vi "setpoint and rotate.vi"(0 "axis 1: sp position °":dbl, 1 "m/c temp setpoint":dbl, 5 "move axis 1":bool, 7 "axis 2: sp position °":dbl, 9 "move axis 2":bool, 11 "error in":errorcluster) -> (4 "Status OUT":T1, 15 "error out":errorcluster)   [LabVIEW 2019]
uses:
  <vilib>/Analysis/NI_AALBase.lvlib
panel:
  out "iterations":i32
  out "standard deviation":dbl format="%0.2f"
  out "mean temperature":dbl format="%0.2f"
  out "m/c temp":dbl
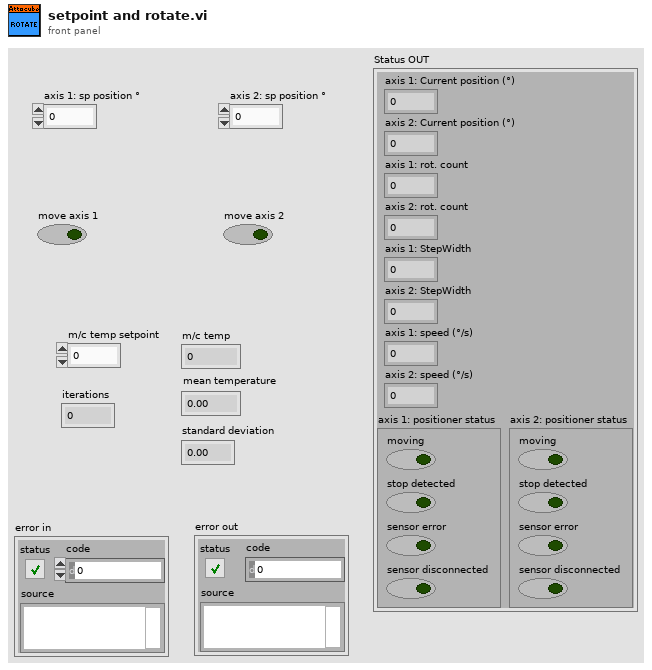
[diagram p1: front panel]
types:
  T1 = cluster{"axis 1: Current position (°)":dbl, "axis 2: Current position (°)":dbl, "axis 1: rot. count":dbl, "axis 2: rot. count":dbl, "axis 1: StepWidth":dbl, "axis 2: StepWidth":dbl, "axis 1: speed (°/s)":dbl, "axis 2: speed (°/s)":dbl, "axis 1: positioner status":cluster{"moving":bool, "stop detected":bool, "sensor error":bool, "sensor disconnected":bool}, "axis 2: positioner status":cluster{"moving":bool, "stop detected":bool, "sensor error":bool, "sensor disconnected":bool}}
  T2 = cluster{"axis 1: Absolute":bool, "axis 2: Absolute":bool, "axis 1: Stop moving":bool, "axis 2: Stop moving":bool, "axis 1: Output":bool, "axis 2: Output":bool, "set static amplitude\nwhen moving":bool}
  T3 = cluster{"axis 1: Amplitude [V]":dbl, "axis 2: Amplitude [V]":dbl, "axis 1: DCLevel [V]":dbl, "axis 2: DCLevel [V]":dbl, "axis 1: Frequency [Hz]":dbl, "axis 2: Frequency [Hz]":dbl, "axis 1: sp position °":dbl, "axis 2: sp position °":dbl, "axis 1: sp rot count":dbl, "axis 2: sp rot count":dbl}
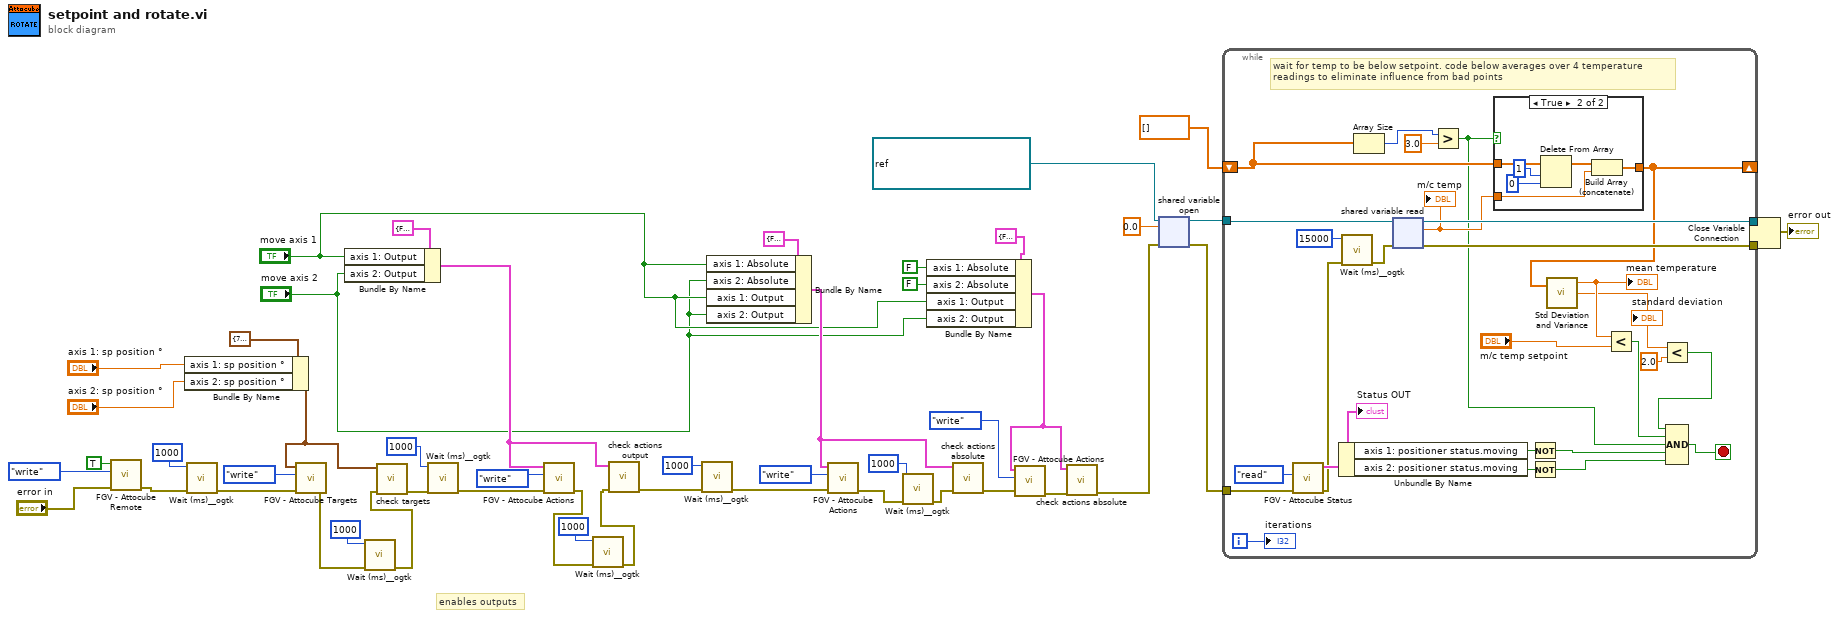
[diagram p0: block diagram]
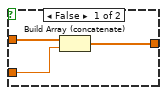
[diagram p2: hidden frame]
diagram:
  # "enables outputs"
  n1 = call "FGV - Attocube Remote.vi"("error in"="error in", "Function"=enum16{"write", "read"}."write", "Attocube Remote"=TRUE) -> ("error out"=w28:errorcluster)  [unwired: 3 in, 1 out]
  n2 = Bundle By Name(cluster=T3 {"axis 1: Amplitude [V]"=70.0, "axis 2: Amplitude [V]"=65.0, "axis 1: DCLevel [V]"=0.0, "axis 2: DCLevel [V]"=0.0, "axis 1: Frequency [Hz]"=3500.0, "axis 2: Frequency [Hz]"=3500.0, "axis 1: sp position °"=230.0, "axis 2: sp position °"=255.0, "axis 1: sp rot count"=0.0, "axis 2: sp rot count"=0.0} ("Targets In"), "axis 1: sp position °"="axis 1: sp position °", "axis 2: sp position °"="axis 2: sp position °") -> (w21:T3)
  n3 = call <userlib>:"Wait (ms)__ogtk.vi"("error in (no error)"=w28, "milliseconds to wait"=u32 1000) -> ("error out"=w27:errorcluster)  [unwired: 8 in, 1 out]
  n4 = call "FGV - Attocube Targets.vi"("error in"=w27, "Function"=enum16{"write", "read"}."write", "Targets In"=w21) -> ("error out"=w19:errorcluster)  [unwired: 3 in, 1 out]
  n5 = Bundle By Name(cluster=T2 {"axis 1: Absolute"=FALSE, "axis 2: Absolute"=FALSE, "axis 1: Stop moving"=FALSE, "axis 2: Stop moving"=FALSE, "axis 1: Output"=FALSE, "axis 2: Output"=FALSE, "set static amplitude\nwhen moving"=FALSE} ("Actions IN"), "axis 1: Output"="move axis 1", "axis 2: Output"="move axis 2") -> (w24:T2)
  n6 = call <userlib>:"Wait (ms)__ogtk.vi"("error in (no error)"=w19, "milliseconds to wait"=u32 1000) -> ("error out"=w18:errorcluster)  [unwired: 8 in, 1 out]
  n7 = call "check targets.vi"("error in"=w18, "Targets In"=w21) -> ("error in 2"=w25:errorcluster)  [unwired: 9 in]
  n8 = call <userlib>:"Wait (ms)__ogtk.vi"("error in (no error)"=w25, "milliseconds to wait"=u32 1000) -> ("error out"=w30:errorcluster)  [unwired: 8 in, 1 out]
  n9 = call "FGV - Attocube Actions.vi"("error in"=w30, "Function"=enum16{"write", "read"}."write", "Actions IN"=w24) -> ("error out"=w16:errorcluster)  [unwired: 3 in, 1 out]
  n10 = call <userlib>:"Wait (ms)__ogtk.vi"("error in (no error)"=w16, "milliseconds to wait"=u32 1000) -> ("error out"=w15:errorcluster)  [unwired: 8 in, 1 out]
  n11 = call "check actions output.vi"("error in"=w15, "Actions IN"=w24) -> ("error in 2"=w23:errorcluster)  [unwired: 9 in]
  n12 = call <userlib>:"Wait (ms)__ogtk.vi"("error in (no error)"=w23, "milliseconds to wait"=u32 1000) -> ("error out"=w32:errorcluster)  [unwired: 8 in, 1 out]
  n13 = Bundle By Name(cluster=T2 {"axis 1: Absolute"=FALSE, "axis 2: Absolute"=FALSE, "axis 1: Stop moving"=FALSE, "axis 2: Stop moving"=FALSE, "axis 1: Output"=FALSE, "axis 2: Output"=FALSE, "set static amplitude\nwhen moving"=FALSE} ("Actions IN"), "axis 1: Absolute"="move axis 1", "axis 2: Absolute"="move axis 2", "axis 1: Output"="move axis 1", "axis 2: Output"="move axis 2") -> (w22:T2)
  n14 = call "FGV - Attocube Actions.vi"("error in"=w32, "Function"=enum16{"write", "read"}."write", "Actions IN"=w22) -> ("error out"=w12:errorcluster)  [unwired: 3 in, 1 out]
  n15 = call <userlib>:"Wait (ms)__ogtk.vi"("error in (no error)"=w12, "milliseconds to wait"=u32 1000) -> ("error out"=w14:errorcluster)  [unwired: 8 in, 1 out]
  n16 = Bundle By Name(cluster=T2 {"axis 1: Absolute"=FALSE, "axis 2: Absolute"=FALSE, "axis 1: Stop moving"=FALSE, "axis 2: Stop moving"=FALSE, "axis 1: Output"=FALSE, "axis 2: Output"=FALSE, "set static amplitude\nwhen moving"=FALSE} ("Actions IN"), "axis 1: Absolute"=FALSE, "axis 2: Absolute"=FALSE, "axis 1: Output"="move axis 1", "axis 2: Output"="move axis 2") -> (w2:T2)
  n17 = call "check actions absolute.vi"("error in"=w14, "Actions IN"=w22) -> ("error in 2"=w11:errorcluster)  [unwired: 9 in]
  n18 = call "FGV - Attocube Actions.vi"("error in"=w11, "Function"=enum16{"write", "read"}."write", "Actions IN"=w2) -> ("error out"=w8:errorcluster)  [unwired: 3 in, 1 out]
  n19 = call "check actions absolute.vi"("error in"=w8, "Actions IN"=w2) -> ("error in 2"=w3:errorcluster)  [unwired: 9 in]
  n20 = shared-variable-open(refnum<k21> "ni.var.psp://housesoftheholy/MNK_18T/MNK_TC_T3" ("shared variable refnum in"), w3, 0.0) -> (w36:refnum<k21>, w37:errorcluster)  [unwired: 1 in]
  n21 = while {
    tunnel: w37 -> [w75]
    tunnel: w36 -> [w72]
    tunnel: [w71] -> w35
    tunnel: [w70] -> w34
    shift-right: [w61] -> _
    shift-left: dbl[] [] -> [w66]
    i -> [w51]
    stop <- w56 stop-if-true
    # "wait for temp to be below setpoint. code below averages over 4 temperature\nreadings to eliminate influence from bad points"
    n22 = call "FGV - Attocube Status.vi"("error in"=w75, "Function"=enum16{"write", "read"}."read") -> ("error out"=w67:errorcluster, "Status OUT"=w77:T1)  [unwired: 4 in]
    "Status OUT" <- w77
    n23 = Unbundle By Name(w77) -> ("axis 1: positioner status.moving"=w74:bool, "axis 2: positioner status.moving"=w73:bool)
    n24 = call <userlib>:"Wait (ms)__ogtk.vi"("error in (no error)"=w67, "milliseconds to wait"=u32 15000) -> ("error out"=w63:errorcluster)  [unwired: 8 in, 1 out]
    n25 = Array Size(array=w66) -> (size(s)=w64:i32)
    n26 = shared-variable-read(w72, w63) -> (w71:refnum<k21>, w70:errorcluster, w62:dbl)  [unwired: 1 out]
    "m/c temp" <- w62
    n27 = Greater?(x=w64, y=3.0) -> (0:w55:bool)
    n28 = case shown="True" w55 {
      tunnel: w66 -> [w80 w86]
      tunnel: [w79 w81] -> w61
      tunnel: w62 -> [w78 w82]
      frame False {
        n29 = Build Array (concatenate)(w80, w78) -> (w79:dbl[])
      }
      frame True {
        n30 = Delete From Array(array=w86, length=1, index=0) -> (array with subset deleted=w83:dbl[])  [unwired: 1 out]
        n31 = Build Array (concatenate)(w83, w82) -> (w81:dbl[])
      }
    }
    n32 = Not(x=w74) -> (.not. x?=w58:bool)
    n33 = Not(x=w73) -> (.not. x?=w57:bool)
    n34 = call <vilib>:"Std Deviation and Variance.vi"("X"=w61) -> ("mean"=w60:dbl, "standard deviation"=w54:dbl)  [unwired: 1 in, 1 out]
    "mean temperature" <- w60
    "standard deviation" <- w54
    n35 = Less?(x=w60, y="m/c temp setpoint") -> (x < y?=w59:bool)
    n36 = Less?(x=w54, y=2.0) -> (x < y?=w52:bool)
    n37 = Compound Arithmetic op=AND(w52, w59, w55, w58, w57) -> (w56:bool)
    "iterations" <- w51
  }
  n38 = Close Variable Connection(8:w34, 11:w35) -> (0:→"error out":errorcluster)
